vi "AverageVorticity.vi"(0 "AVG#":i32, 1 "step vort":i32, 3 "v average":i32, 5 "Mean/Median":u16(ring) items=["Median", "Mean"], 7 "No Mask?":bool, 9 "Velocity field":csg[][][](array[numeric]), 11 "Values":T2, 12 "y scale":sgl, 13 "vort min val":dbl, 14 "Cursor positions":T1[](array[typedef])) -> (6 "Energy loss v time in window":dbl[](graph), 8 "KE vs time":dbl[](array[numeric]), 10 "Average vorticity v time rad/s":dbl[][](graph), 15 "All vorticity":dbl[][][](array[numeric]))   [LabVIEW 2022 SP3]
uses:
  VPIParams.ctl
  <vilib>/Utility/miscctls.llb/LVPointDoubleTypeDef.ctl
  <vilib>/Analysis/NI_AALBase.lvlib
panel:
  out "SD vorticity":dbl[](graph)
  out "mean vs time":dbl[][](graph)
  out "energy loss":dbl[][](graph)
  out "vorticity":dbl[][](graph)
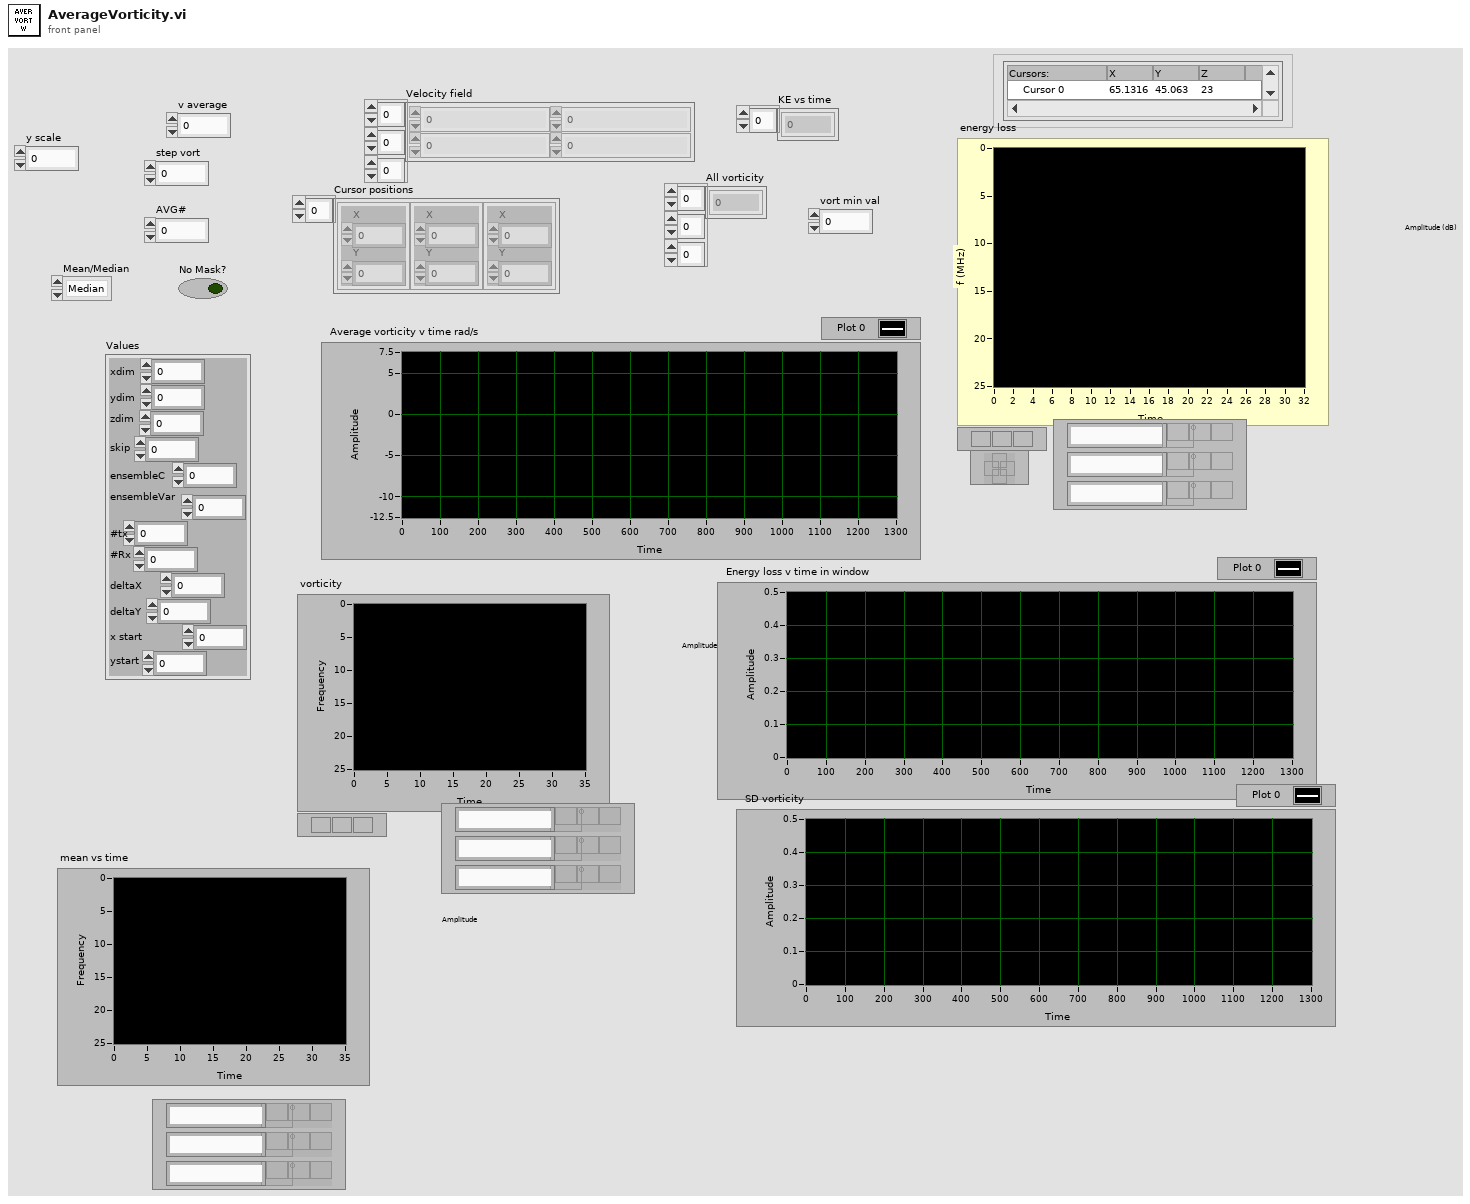
[diagram p1: front panel]
types:
  T1 = typedef "LVPointDoubleTypeDef.ctl" = cluster{"X":dbl, "Y":dbl}
  T2 = typedef "VPIParams.ctl" = cluster{"xdim":dbl, "ydim":dbl, "zdim":dbl, "skip":dbl, "ensembleC":dbl, "ensembleVar\n":dbl, "#tx":dbl, "#Rx":dbl, "deltaX":dbl, "deltaY":dbl, "x start":dbl, "ystart":dbl}
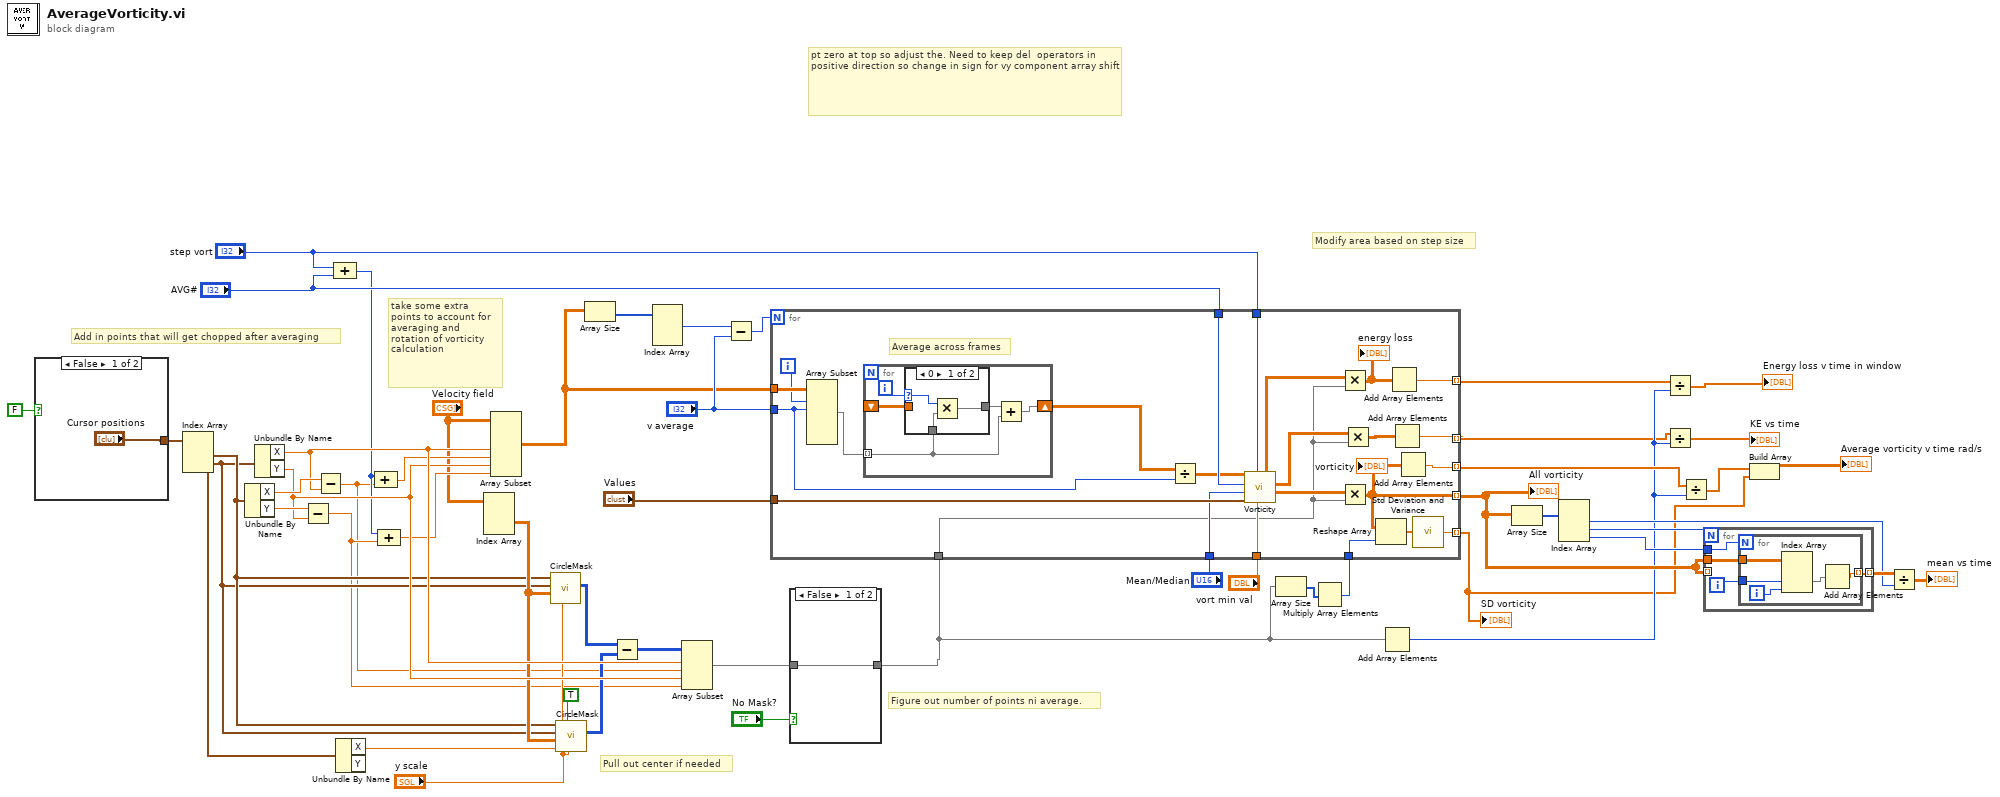
[diagram p0: block diagram]
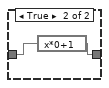
[diagram p2: hidden frame]
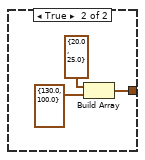
[diagram p3: hidden frame]
diagram:
  # "take some extra points to account for averaging and rotation of vorticity calculation"
  # "Figure out number of points ni average."
  # "Pull out center if needed"
  # "Add in points that will get chopped after averaging"
  # "Modify area based on step size"
  # "pt zero at top so adjust the. Need to keep del  operators in positive direction so change in sign for vy component array shift"
  n1 = case shown="False" FALSE {
    tunnel: ["Cursor positions" w55] -> w37
    frame False {
    }
    frame True {
      n2 = Build Array(T1 {"X"=20.0, "Y"=25.0} ("Cursor.Cursor Position"), T1 {"X"=130.0, "Y"=100.0} ("Cursor.Cursor Position")) -> (w55:T1[])
    }
  }
  n3 = Index Array(array=w37) -> (element #1=w20:T1, element #2=w19:T1, element #3=w18:T1)  [unwired: 3 in]
  n4 = Unbundle By Name(w20) -> ("X"=w51:dbl, "Y"=w50:dbl)
  n5 = Unbundle By Name(w19) -> ("X"=w36:dbl, "Y"=w34:dbl)
  n6 = Subtract(x=w50, y=w34) -> (x-y=w11:dbl)
  n7 = Subtract(x=w51, y=w36) -> (x-y=w10:dbl)
  n8 = Compound Arithmetic op=ADD("step vort", "AVG#") -> (w14:i32)
  n9 = Unbundle By Name(w18) -> ("X"=w17:dbl)  [unwired: 1 out]
  n10 = Compound Arithmetic op=unknown(w14, w10) -> (w35:dbl)
  n11 = Compound Arithmetic op=unknown(w14, w11) -> (w33:dbl)
  n12 = Index Array(array="Velocity field") -> (element=w29:csg[][])  [unwired: 3 in]
  n13 = Array Subset(array="Velocity field", index (dim 1)=w36, length (dim 1)=w35, index (dim 2)=w34, length (dim 2)=w33) -> (w27:csg[][][])  [unwired: 2 in]
  n14 = call "CircleMask.vi"("y scale"="y scale", "Array in"=w29, "Cursor 1"=w19, "Cursor 0"=w20) -> ("Array 3"=w23:i16[][])  [unwired: 6 in, 1 out]
  n15 = call "CircleMask.vi"("y scale"="y scale", "Radius Override"=TRUE, "Force radius"=w17, "Array in"=w29, "Cursor 1"=w19, "Cursor 0"=w20) -> ("Array 3"=w22:i16[][])  [unwired: 4 in, 1 out]
  n16 = Array Size(array=w27) -> (size(s)=w52:i32[])
  n17 = Subtract(x=w23, y=w22) -> (x-y=w21:i16[][])
  n18 = Index Array(array=w52) -> (element #1=w47:i32)  [unwired: 3 in, 2 out]
  n19 = Array Subset(array=w21, index (row)=w36, length (row)=w10, index (col)=w34, length (col)=w11) -> (w13:i16[][])
  n20 = Subtract(x=w47, y="v average") -> (x-y=w46:i32)
  n21 = case shown="False" "No Mask?" {
    tunnel: [w58 w60] -> w6
    tunnel: w13 -> [w58 w59]
    frame False {
    }
    frame True {
      n22 = expression code="x*0+1"(w59) -> (w60:i16[][])
    }
  }
  n23 = Array Size(array=w6) -> (size(s)=w5:i32[])
  n24 = Multiply Array Elements(1:w5) -> (0:w4:i32)
  n25 = for {
    N: w46 -> [_]
    tunnel: "Values" -> [w84]
    tunnel: "vort min val" -> [w83]
    tunnel: "step vort" -> [w82]
    tunnel: w27 -> [w81]
    tunnel: "v average" -> [w78]
    tunnel: [w61] -> w40 mode=indexing
    tunnel: [w79] -> w41 mode=indexing
    tunnel: "AVG#" -> [w76]
    tunnel: "Mean/Median" -> [w75]
    tunnel: [w74] -> w42 mode=indexing
    tunnel: [w70] -> w24 mode=indexing
    tunnel: w6 -> [w67]
    tunnel: [w63] -> w1 mode=indexing
    tunnel: w4 -> [w62]
    i -> [w80]
    # "Average across frames"
    n26 = Array Subset(array=w81, index (dim 0)=w80, length (dim 0)=w78) -> (w73:csg[][][])  [unwired: 4 in]
    n27 = for {
      tunnel: w73 -> [w85] mode=indexing
      shift-right: [w89] -> w77
      shift-left: _ -> [w87]
      i -> [w86]
      n28 = case shown="0" w86 {
        selector: w86 -> [w92 _]
        tunnel: [w91 w93] -> w88
        tunnel: w87 -> [_ w93]
        tunnel: w85 -> [w90 _]
        frame 0 {
          n29 = Multiply(x=w92, y=w90) -> (x*y=w91:csg[][])
        }
        frame 1, Default {
        }
      }
      n30 = Add(x=w88, y=w85) -> (x+y=w89:csg[][])
    }
    n31 = Divide(x=w77, y=w78) -> (x/y=w72:csg[][])
    n32 = call "Vorticity.vi"("vort min val"=w83, "step vort"=w82, "Values"=w84, "Mean/Median"=w75, "AVG #"=w76, "Vector out"=w72) -> ("vorticity rad/s"=w68:dbl[][], "KE"=w69:dbl[][], "EL mW/m"=w65:dbl[][])  [unwired: 2 in, 1 out]
    n33 = Multiply(x=w65, y=w67) -> (x*y=w66:dbl[][])
    "energy loss" <- w66
    n34 = Multiply(x=w68, y=w67) -> (x*y=w61:dbl[][])
    "vorticity" <- w61
    n35 = Multiply(x=w69, y=w67) -> (x*y=w71:dbl[][])
    n36 = Reshape Array(w61, w62) -> (w64:dbl[])
    n37 = Add Array Elements(numeric array=w66) -> (sum=w79:dbl)
    n38 = Add Array Elements(numeric array=w71) -> (sum=w70:dbl)
    n39 = Add Array Elements(numeric array=w61) -> (sum=w74:dbl)
    n40 = call <vilib>:"Std Deviation and Variance.vi"("X"=w64) -> ("standard deviation"=w63:dbl)  [unwired: 1 in, 2 out]
  }
  "All vorticity" <- w40
  "SD vorticity" <- w1
  n41 = Add Array Elements(numeric array=w6) -> (sum=w25:i16)
  n42 = Array Size(array=w40) -> (size(s)=w45:i32[])
  n43 = Index Array(array=w45) -> (element #1=w26:i32, element #2=w39:i32, element #3=w38:i32)  [unwired: 3 in]
  n44 = Divide(x=w41, y=w25) -> (x/y=→"Energy loss v time in window":dbl[])
  n45 = Divide(x=w24, y=w25) -> (x/y=→"KE vs time":dbl[])
  n46 = Divide(x=w42, y=w25) -> (x/y=w3:dbl[])
  n47 = for {
    N: w39 -> [_]
    tunnel: w40 -> [_] mode=indexing
    tunnel: w40 -> [w97]
    tunnel: w38 -> [w96]
    tunnel: [w94] -> w31 mode=indexing
    i -> [w95]
    n48 = for {
      N: w96 -> [_]
      tunnel: w97 -> [w102]
      tunnel: w95 -> [w100]
      tunnel: [w98] -> w94 mode=indexing
      i -> [w101]
      n49 = Index Array(array=w102, index (dim 1)=w100, index (dim 2)=w101) -> (element=w99:dbl[])  [unwired: 1 in]
      n50 = Add Array Elements(numeric array=w99) -> (sum=w98:dbl)
    }
  }
  n51 = Build Array(w3, w1) -> (→"Average vorticity v time rad/s":dbl[][])
  n52 = Divide(x=w31, y=w26) -> (x/y=→"mean vs time":dbl[][])
